vi "FunnelGenerateFillPath.vi"(9 "Curve 2":cluster{"X":dbl, "Y":dbl}[](array[cluster])=[{"X"=33.345441, "Y"=13.920885}, {"X"=33.82141111495116, "Y"=14.019594874530428}, {"X"=34.29231286175806, "Y"=14.130238690458299}, {"X"=34.75675225244177, "Y"=14.256098736288504}, {"X"=35.2133352990233, "Y"=14.40045730052592}, {"X"=35.660668013523654, "Y"=14.566596671675429}, {"X"=36.09735640796393, "Y"=14.757799138241921}, {"X"=36.52200649436513, "Y"=14.977346988730275}, {"X"=36.933224284748306, "Y"=15.22852251164538}, {"X"=37.329615791134486, "Y"=15.51460799549211}, {"X"=37.7097870255447, "Y"=15.838885728775356}, {"X"=38.072343999999994, "Y"=16.204638}], 10 "Curve 1":cluster{"X":dbl, "Y":dbl}[](array[cluster])=[{"X"=38.027750999999995, "Y"=11.610882}, {"X"=37.62650350187828, "Y"=11.870325879038317}, {"X"=37.219808535687434, "Y"=12.118738800901575}, {"X"=36.80785412096168, "Y"=12.356501510894063}, {"X"=36.39082827723516, "Y"=12.583994754320061}, {"X"=35.968919024042066, "Y"=12.801599276483847}, {"X"=35.5423143809166, "Y"=13.009695822689707}, {"X"=35.111202367392934, "Y"=13.208665138241921}, {"X"=34.67577100300526, "Y"=13.398887968444779}, {"X"=34.236208307287754, "Y"=13.580745058602556}, {"X"=33.792702299774604, "Y"=13.754617154019535}, {"X"=33.345441, "Y"=13.920885}], 11 "Bottom Segments":i32=3) -> (3 "Funnel Path":cluster{dbl, dbl}[](array[cluster]))   [LabVIEW 2019]
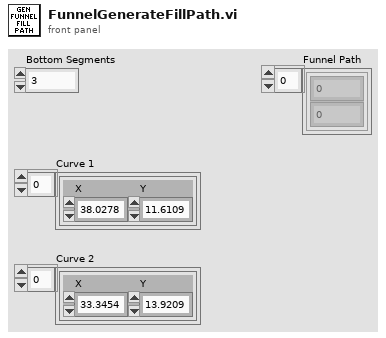
[diagram p1: front panel]
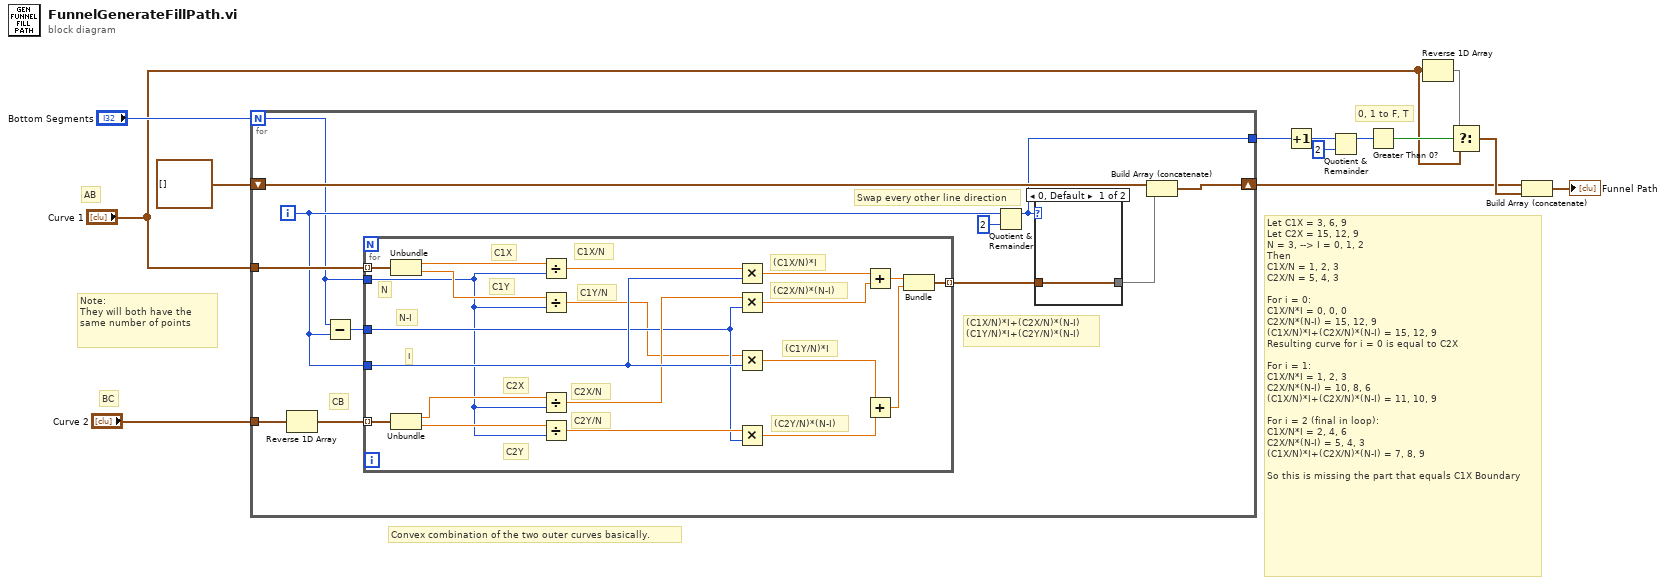
[diagram p0: block diagram]
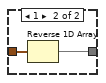
[diagram p2: hidden frame]
diagram:
  # "Convex combination of the two outer curves basically."
  # "BC"
  # "AB"
  # "0, 1 to F, T"
  # "Let C1X = 3, 6, 9\nLet C2X = 15, 12, 9\nN = 3, --> I = 0, 1, 2\nThen \nC1X/N = 1, 2, 3\nC2X/N = 5, 4, 3\n\nFor i = 0:\nC1X/N*I = 0, 0, 0\nC2X/N*(N-I) = 15, 12, 9\n(C1X/N)*I+(C2X/N)*(N-I) = 15, 12, 9\nResulting curve for i = 0 is equal to C2X\n\nFor i = 1:\nC1X/N*I = 1, 2, 3\nC2X/N*(N-I) = 10, 8, 6\n(C1X/N)*I+(C2X/N)*(N-I) = 11, 10, 9\n\nFor i = 2 (final in loop):\nC1X/N*I = 2, 4, 6\nC2X/N*(N-I) = 5, 4, 3\n(C1X/N)*I+(C2X/N)*(N-I) = 7, 8, 9\n\nSo this is missing the part that equals C1X Boundary"
  # "Note:\nThey will both have the same number of points"
  n1 = for {
    N: "Bottom Segments" -> [w14]
    tunnel: "Curve 2" -> [w21]
    shift-right: [w17] -> w3
    shift-left: cluster{dbl, dbl}[] [] -> [w24]
    tunnel: "Curve 1" -> [w20]
    tunnel: [w15] -> w10
    i -> [w19]
    # "CB"
    # "Swap every other line direction"
    # "(C1X/N)*I+(C2X/N)*(N-I)\n(C1Y/N)*I+(C2Y/N)*(N-I)"
    n2 = Reverse 1D Array(array=w21) -> (reversed array=w23:cluster{"X":dbl, "Y":dbl}[])
    n3 = Subtract(x=w14, y=w19) -> (x-y=w25:i32)
    n4 = for {
      tunnel: w20 -> [w48] mode=indexing
      tunnel: w23 -> [w47] mode=indexing
      tunnel: w19 -> [w43]
      tunnel: w25 -> [w38]
      tunnel: [w33] -> w18 mode=indexing
      tunnel: w14 -> [w32]
      # "C2Y"
      # "I"
      # "N"
      # "N-I"
      # "(C2Y/N)*(N-I)"
      # "C2Y/N"
      # "(C2X/N)*(N-I)"
      # "C2X/N"
      # "C2X"
      # "(C1Y/N)*I"
      # "C1Y/N"
      # "C1Y"
      # "(C1X/N)*I"
      # "C1X/N"
      # "C1X"
      n5 = Unbundle(w48) -> ("X"=w46:dbl, "Y"=w44:dbl)
      n6 = Unbundle(w47) -> ("X"=w42:dbl, "Y"=w41:dbl)
      n7 = Divide(x=w46, y=w32) -> (x/y=w45:dbl)
      n8 = Divide(x=w44, y=w32) -> (x/y=w30:dbl)
      n9 = Divide(x=w42, y=w32) -> (x/y=w40:dbl)
      n10 = Divide(x=w41, y=w32) -> (x/y=w39:dbl)
      n11 = Multiply(x=w45, y=w43) -> (x*y=w37:dbl)
      n12 = Multiply(x=w40, y=w38) -> (x*y=w36:dbl)
      n13 = Multiply(x=w30, y=w43) -> (x*y=w35:dbl)
      n14 = Multiply(x=w39, y=w38) -> (x*y=w29:dbl)
      n15 = Add(x=w37, y=w36) -> (x+y=w34:dbl)
      n16 = Add(x=w35, y=w29) -> (x+y=w31:dbl)
      n17 = Bundle(w34, w31) -> (w33:cluster{dbl, dbl})  [unwired: 1 in]
    }
    n18 = Quotient & Remainder(x=w19, y=2) -> (x-y*floor(x/y)=w15:i32)  [unwired: 1 out]
    n19 = case shown="0, Default" w15 {
      tunnel: w18 -> [w26 w28]
      tunnel: [w26 w27] -> w16
      frame 0, Default {
      }
      frame 1 {
        n20 = Reverse 1D Array(array=w28) -> (reversed array=w27:cluster{dbl, dbl}[])
      }
    }
    n21 = Build Array (concatenate)(w24, w16) -> (w17:cluster{dbl, dbl}[])
  }
  n22 = Increment(x=w10) -> (x+1=w8:i32)
  n23 = Quotient & Remainder(x=w8, y=2) -> (x-y*floor(x/y)=w7:i32)  [unwired: 1 out]
  n24 = Greater Than 0?(x=w7) -> (x > 0?=w6:bool)
  n25 = Reverse 1D Array(array="Curve 1") -> (reversed array=w5:cluster{"X":dbl, "Y":dbl}[])
  n26 = Select(t=w5, s=w6, f="Curve 1") -> (s? t:f=w4:cluster{"X":dbl, "Y":dbl}[])
  n27 = Build Array (concatenate)(w3, w4) -> (→"Funnel Path":cluster{"X":dbl, "Y":dbl}[])
